vi "引用測試5.vi"() -> ()   [LabVIEW 2015]
uses:
  <vilib>/vision/Measure.llb/Edge Options.ctl
  <vilib>/vision/Measure.llb/Edge Polarity.ctl
  <vilib>/userdefined/High Color/IMAQdx.ctl
  <vilib>/vision/driver/NI_Vision_Acquisition_Software.lvlib
  <vilib>/vision/NI_Vision_Development_Module.lvlib
panel:
  in  "Tab Control":T1(tab)
  in  "邊":T2(ring)
  out "Line Data":cluster{"X":sgl, "Y":sgl, "T":sgl}
  in  "圓":enum16{"Inner to Outer", "Outer to Inner"}(ring)
  out "Ellipse":T3 {"Minor Axis"."Point 2"."Y" format="%.2f"; "Minor Axis"."Point 2"."X" format="%.2f"; "Minor Axis"."Point 1"."Y" format="%.2f"; "Minor Axis"."Point 1"."X" format="%.2f"; "Major Axis"."Point 2"."Y" format="%.2f"; "Major Axis"."Point 2"."X" format="%.2f"; "Major Axis"."Point 1"."Y" format="%.2f"; "Major Axis"."Point 1"."X" format="%.2f"; "Center"."Y" format="%.2f"; "Center"."X" format="%.2f"}
  in  "線":enum16{"Start to End", "End to Start"}(ring)
  out "Location (Pixel)":cluster{"X":sgl, "Y":sgl}
  in  "DieArea":i32=100 min=10
  in  "ShowData":bool
  in  "抓寬度(方向)":T4(ring)=enum."Horizon(Outer to Inner)"
  in  "Settings":T5={"Contrast"=40, "Filter width"=4, "Steepness"=2, "Subsampling Ratio"=5, "Show Search Area"=FALSE, "Show Search Lines"=FALSE, "Show Edges Found"=FALSE, "Show Result"=TRUE}
  out "Distance":sgl
  in  "繪圖":bool
  in  "繪圖ROI資料":T6=enum."Set Data"
  out "Line Profile":T7(graph)
  in  "Session In":T8="cam1"
  in  "Numeric":i32
  in  "重新開圖":bool
  in  "開圖":bool
  in  "動作":enum16{"什麼也不做", "抓邊", "看灰階", "分析光源均勻度", "抓寬度"}(ring)
  out "Mean":sgl format="%#.2f"
  out "Histogram":T9(graph)
  in  "取像":bool
  in  "Edge Options":T10={"Edge Polarity"=0, "Kernel Size"=3, "Width"=3, "Minimum Edge Strength"=10.0, "Interpolation Type"=enum."Bilinear Fixed", "Data Processing Method"=enum."Average"} {"Edge Polarity" items=["All Edges", "Rising Edges", "Falling Edges"]; "Minimum Edge Strength" format="%.2f"; "Width" step=2; "Kernel Size" step=2}
  out "error out":errorcluster
  out "Gradient Information":dbl[][](graph)
  in  "Process":T12(ring)
  in  "Gap":i32=10 min=1 max=300
  in  "stop":bool
  out "Image":T13(plugin-control)
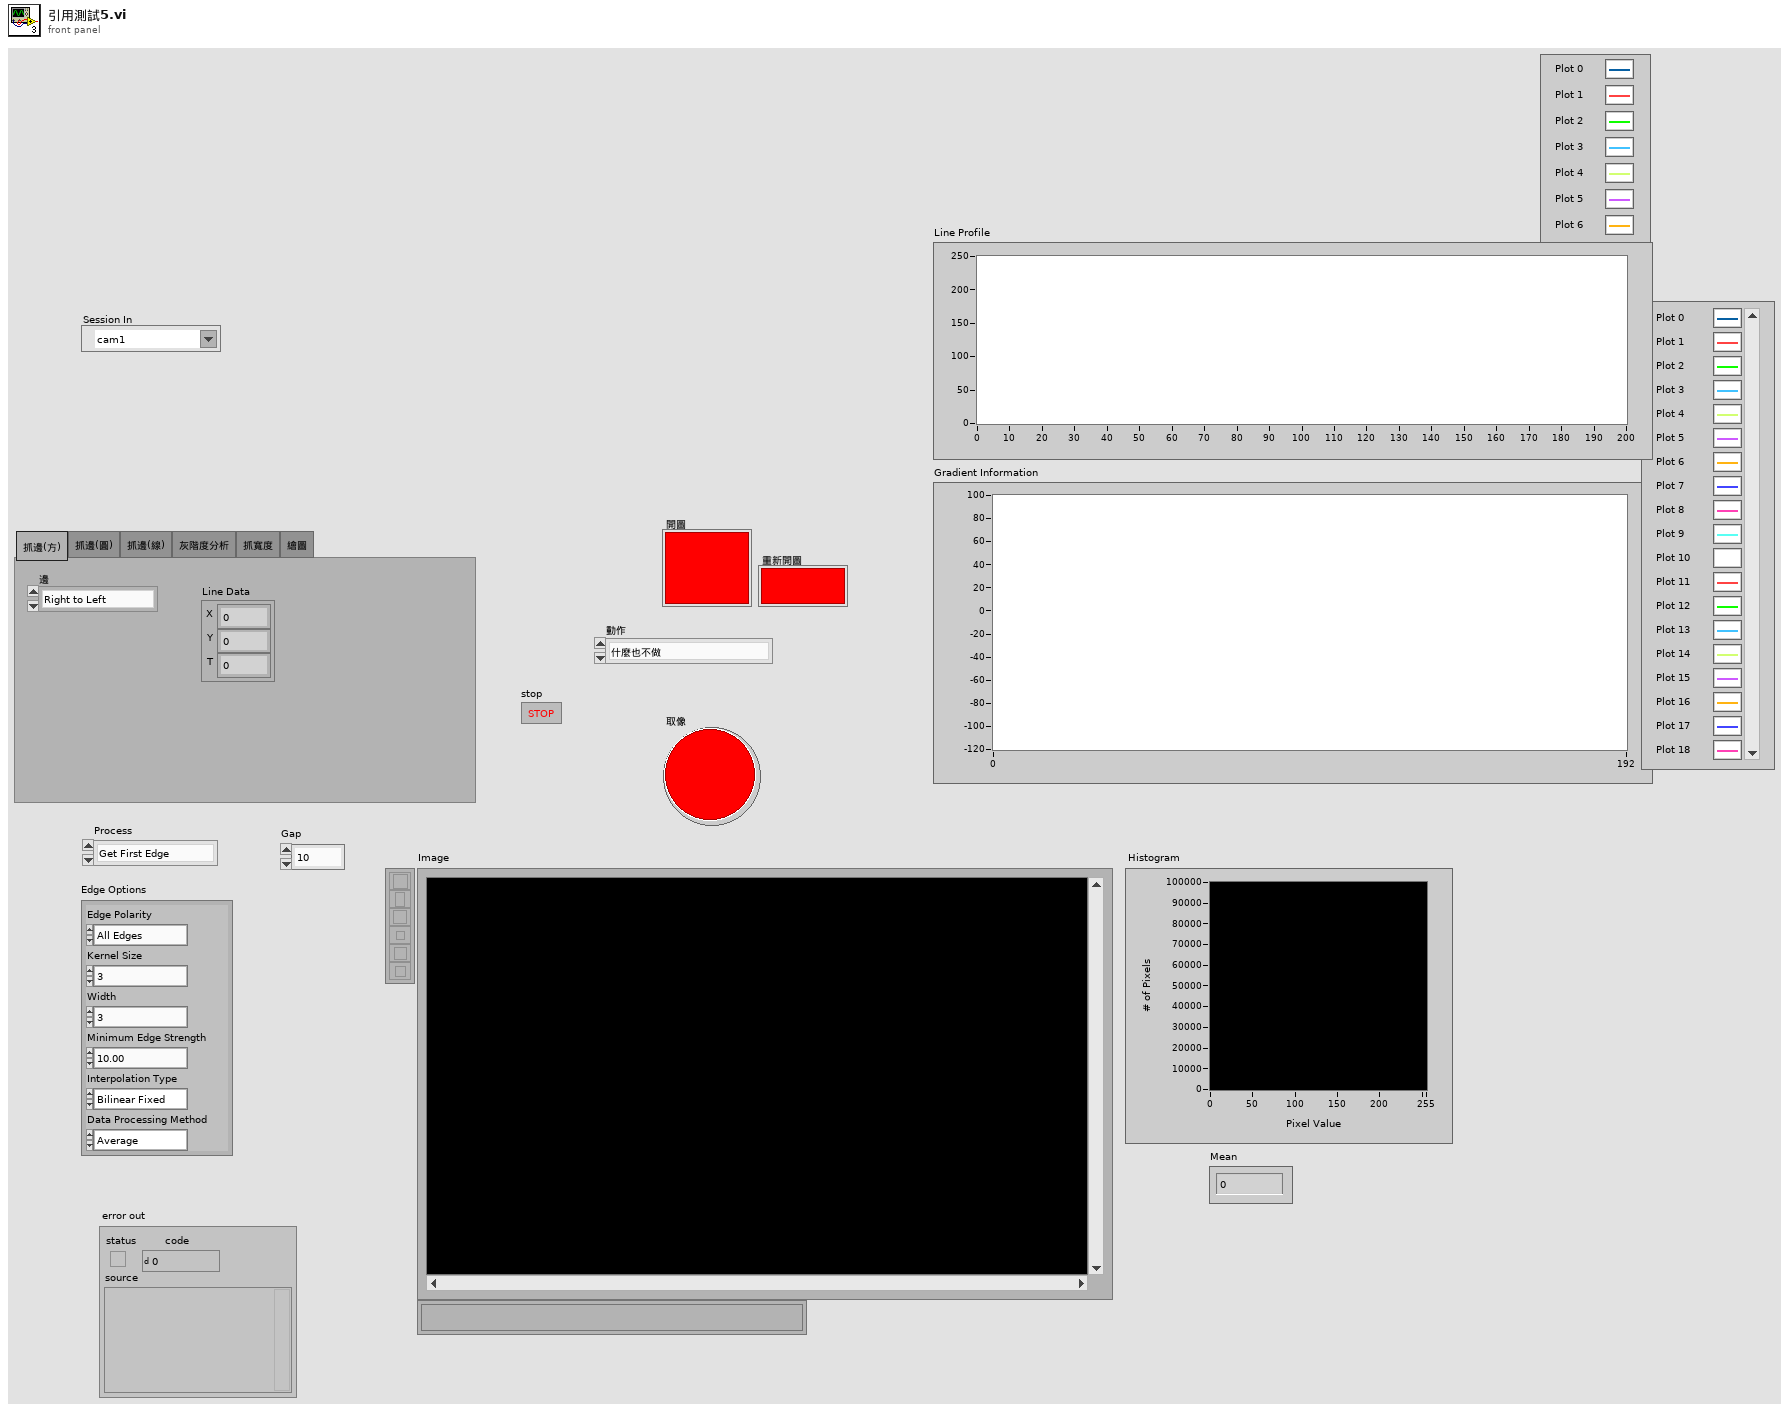
[diagram p1: front panel]
types:
  T1 = enum32{"抓邊(方)", "抓邊(圓)", "抓邊(線)", "灰階度分析", "抓寬度", "繪圖"}
  T2 = enum16{"Right to Left", "Left  to Right", "Up to Down", "Down to Up"}
  T3 = cluster{"Center":cluster{"X":sgl, "Y":sgl}, "Major Axis":cluster{"Point 1":cluster{"X":sgl, "Y":sgl}, "Point 2":cluster{"X":sgl, "Y":sgl}}, "Minor Axis":cluster{"Point 1":cluster{"X":sgl, "Y":sgl}, "Point 2":cluster{"X":sgl, "Y":sgl}}}
  T4 = enum16{"Horizon(Inner to Outer)", "Horizon(Outer to Inner)", "Vertical (Inner to Outer)", "Vertical(Outer to Inner)"}
  T5 = cluster{"Contrast":i32, "Filter width":i32, "Steepness":i32, "Subsampling Ratio":u32, "Show Search Area":bool, "Show Search Lines":bool, "Show Edges Found":bool, "Show Result":bool}
  T6 = typedef "Action_Data.ctl" = enum16{"Initialize", "Get Data", "Set Data", "Delete Data", "Idle"}
  T7 = cluster{"x0":sgl, "dx":sgl, "Pixels Line":sgl[]}[]
  T8 = typedef "IMAQdx.ctl" = refnum<k21>
  T9 = cluster{"Starting Value":sgl, "Incremental Value":sgl, "Histogram":u32[]}
  T10 = typedef "Edge Options.ctl" = cluster{"Edge Polarity":T11, "Kernel Size":u32, "Width":u32, "Minimum Edge Strength":sgl, "Interpolation Type":enum32{"Zero Order", "Bilinear", "Quadratic", "Cubic", "Bilinear Fixed"}, "Data Processing Method":enum32{"Average", "Median"}}
  T11 = typedef "Edge Polarity.ctl" = u32
  T12 = enum16{"Get First Edge", "Get First + Last Edge", "Get All Edges", "Get Best Edge"}
  T13 = typedef "IMAQ Image.ctl" = refnum<image>
  T14 = typedef "IMAQ Rectangle" = cluster{"Left":i32, "Top":i32, "Right":i32, "Bottom":i32, "Rotation":dbl}
  T15 = typedef "ROI Descriptor" = cluster{"Global Rectangle":i32[], "Contours":cluster{"ID":enum32{"External", "Internal"}, "Type":u32, "Coordinates":i32[]}[]}
  T16 = cluster{"Origin":cluster{"X":sgl, "Y":sgl}, "Angle (deg)":sgl, "Axis Reference":u32}
  T17 = typedef "Image Type" = u32
  T18 = cluster{"Global Rectangle":i32[], "Contours":cluster{"Contour Type":u32, "ROI Type":u32, "Points":i32[]}[]}
  T19 = cluster{"Contour Type":u32, "ROI Type":u32, "Points":i32[]}[]
  T20 = cluster{"Contour Type":u32, "ROI Type":u32, "Points":i32[]}
  T21 = enum32{"Zero Order", "Bilinear", "Quadratic", "Cubic", "Bilinear Fixed"}
  T22 = cluster{"邊":enum16{"Right to Left", "Left  to Right", "Up to Down", "Down to Up"}, "動作":enum16{"什麼也不做", "抓邊", "看灰階", "分析光源均勻度", "抓寬度"}, "圓":enum16{"Inner to Outer", "Outer to Inner"}, "Process":enum16{"Get First Edge", "Get First + Last Edge", "Get All Edges", "Get Best Edge"}, "ROI Type":u32, i32, i32, i32, i32, "Gap":i32, i32, i32, i32, i32, "Edge Polarity":T11, "Kernel Size":u32, "Width":u32, "Minimum Edge Strength":sgl, "Interpolation Type":enum32{"Zero Order", "Bilinear", "Quadratic", "Cubic", "Bilinear Fixed"}, "Data Processing Method":enum32{"Average", "Median"}, "DieArea":i32, "ShowData":bool, "線":enum16{"Start to End", "End to Start"}, "抓寬度(方向)":enum16{"Horizon(Inner to Outer)", "Horizon(Outer to Inner)", "Vertical (Inner to Outer)", "Vertical(Outer to Inner)"}, "Contrast":i32, "Filter width":i32, "Steepness":i32, "Subsampling Ratio":u32, "Show Search Area":bool, "Show Search Lines":bool, "Show Edges Found":bool, "Show Result":bool, bool}
  T23 = cluster{"邊":bool, "動作":bool, "圓":bool, "Process":bool, "ROI Type":bool, bool, bool, bool, bool, "Gap":bool, bool, bool, bool, bool, "Edge Polarity":bool, "Kernel Size":bool, "Width":bool, "Minimum Edge Strength":bool, "Interpolation Type":bool, "Data Processing Method":bool, "DieArea":bool, "ShowData":bool, "線":bool, "抓寬度(方向)":bool, "Contrast":bool, "Filter width":bool, "Steepness":bool, "Subsampling Ratio":bool, "Show Search Area":bool, "Show Search Lines":bool, "Show Edges Found":bool, "Show Result":bool, bool}
  T24 = cluster{"Base Reference":cluster{"Origin":cluster{"X":sgl, "Y":sgl}, "Angle (deg)":sgl, "Axis Reference":u32}, "Base Reference":cluster{"Origin":cluster{"X":sgl, "Y":sgl}, "Angle (deg)":sgl, "Axis Reference":u32}}
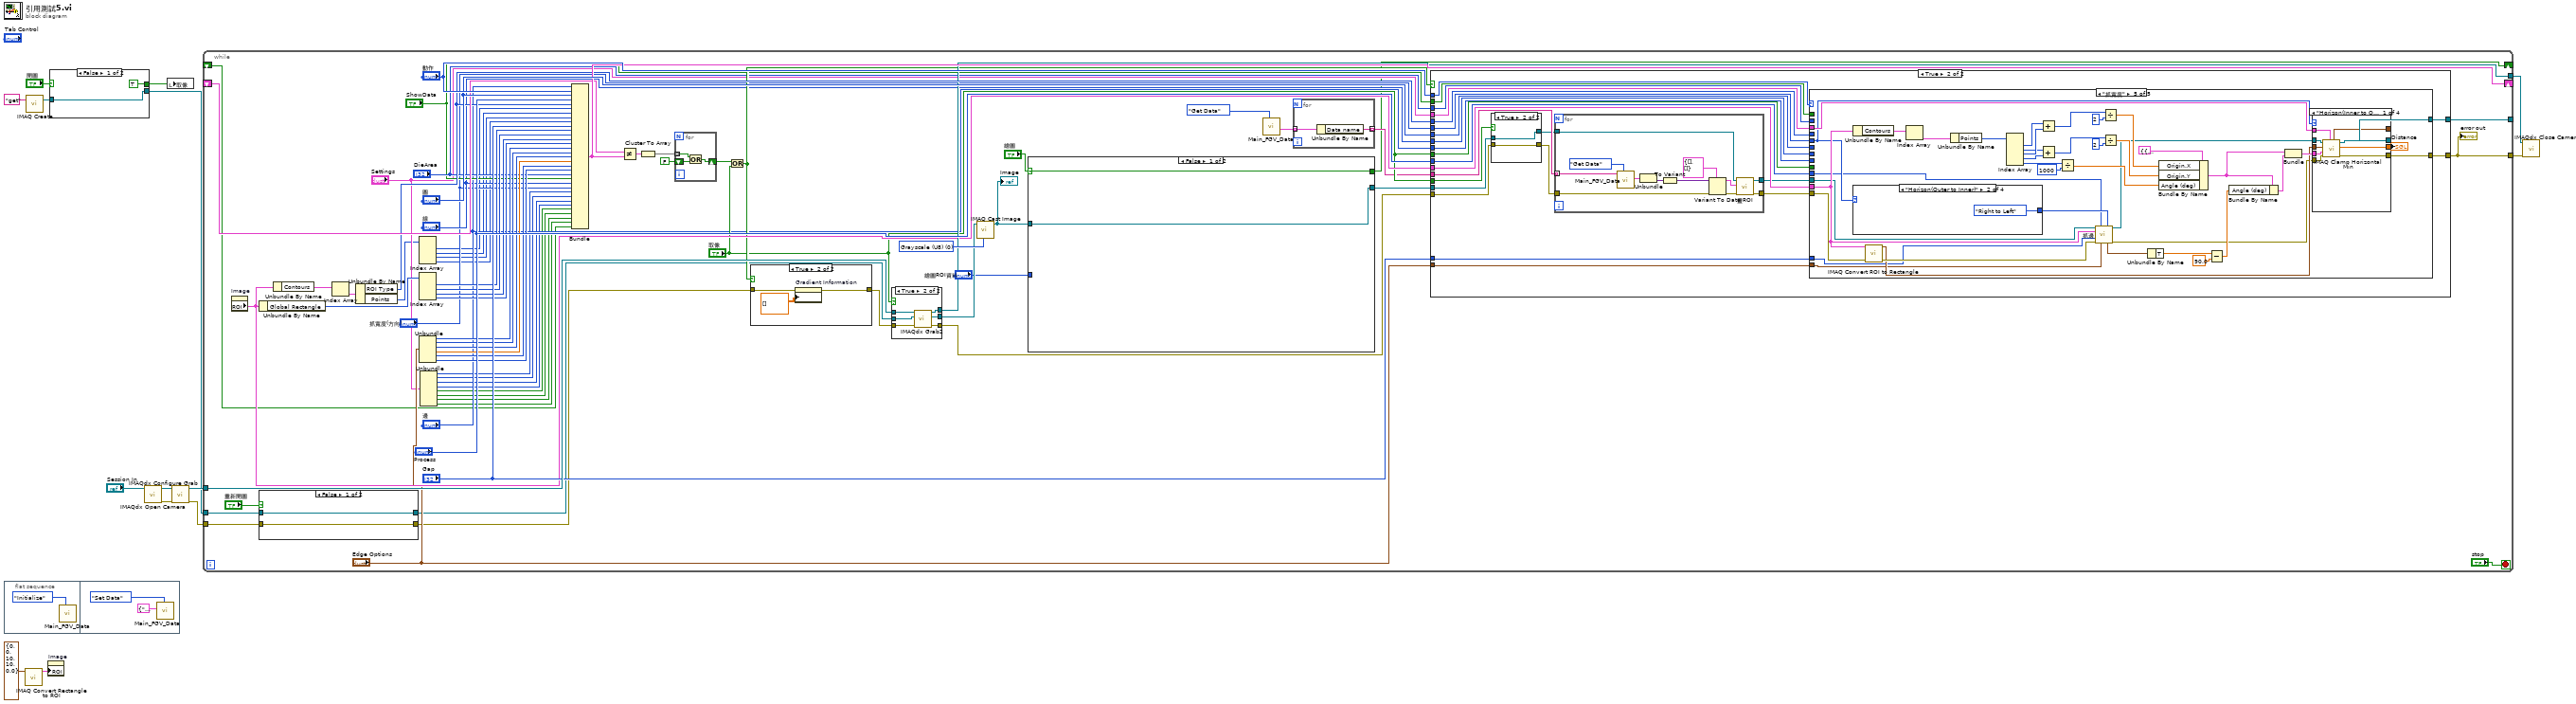
[diagram p0: block diagram]
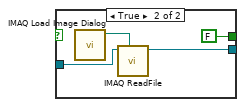
[diagram p2: hidden frame]
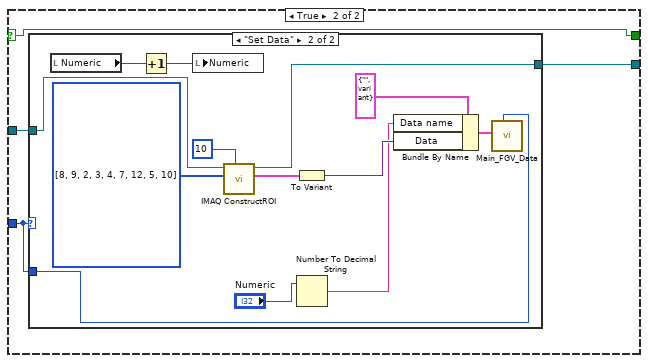
[diagram p3: hidden frame]
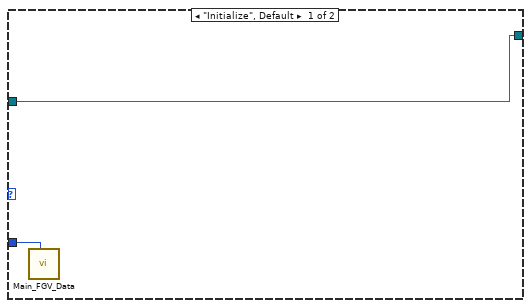
[diagram p4: hidden frame]
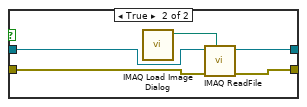
[diagram p5: hidden frame]
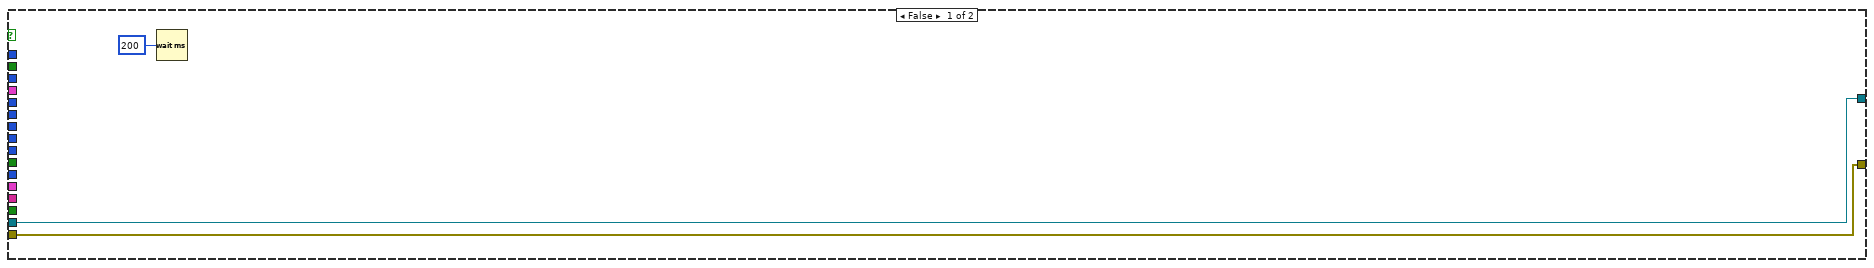
[diagram p7: hidden frame]
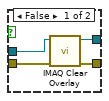
[diagram p8: hidden frame]
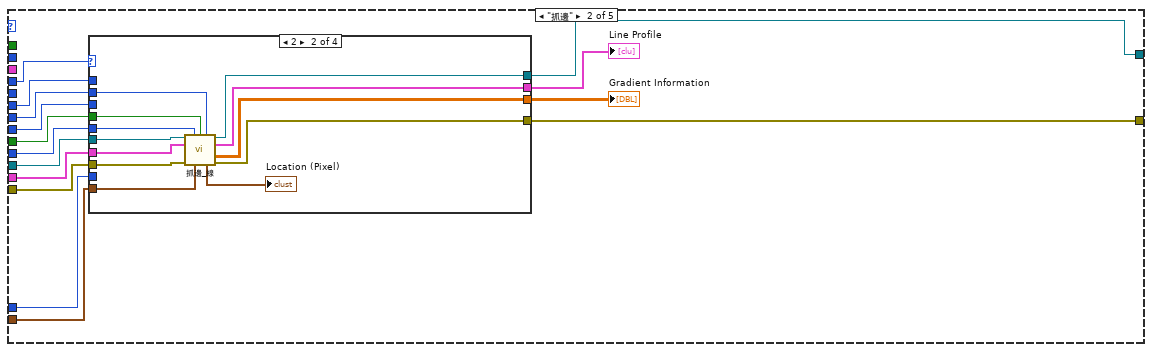
[diagram p10: hidden frame]
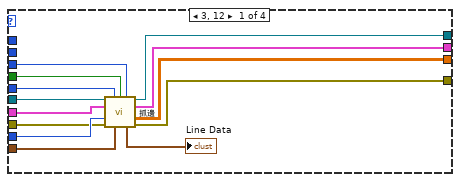
[diagram p11: hidden frame]
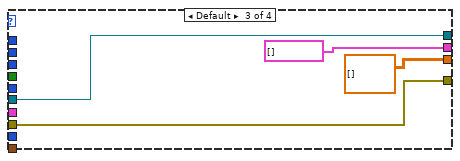
[diagram p12: hidden frame]
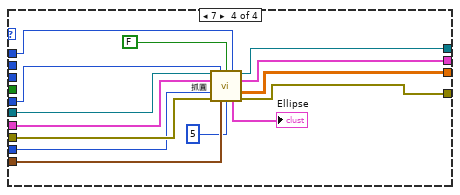
[diagram p13: hidden frame]
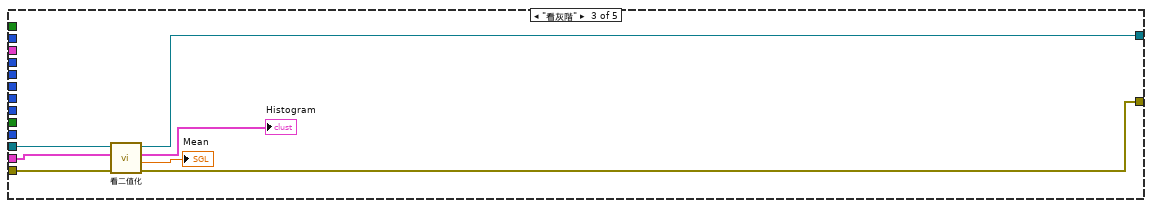
[diagram p14: hidden frame]
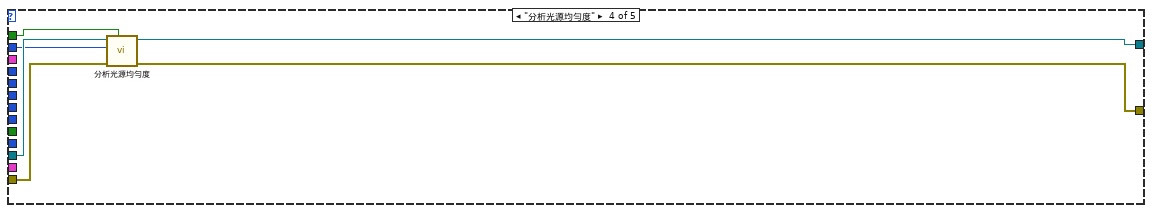
[diagram p15: hidden frame]
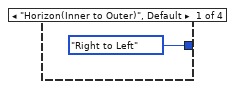
[diagram p16: hidden frame]
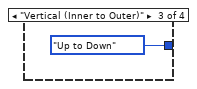
[diagram p17: hidden frame]
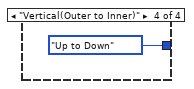
[diagram p18: hidden frame]
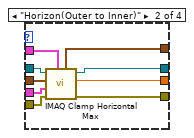
[diagram p19: hidden frame]
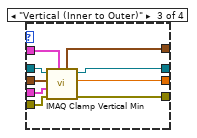
[diagram p20: hidden frame]
diagram:
  n1 = flat-sequence {
    frame #0 {
      n2 = call "Main_FGV_Data.vi"("Action_Data"=Action_Data."Initialize") -> ()  [unwired: 9 in, 2 out]
    }
    frame #1 {
      n3 = call "Main_FGV_Data.vi"("Action_Data"=Action_Data."Set Data", "Data In"=cluster{"Data name":string, "Data":variant} {"Data name"="Oringal", "Data"=variant(cluster{"Global Rectangle":i32[], "Contours":cluster{"ID":enum32{"External", "Internal"}, "Type":u32, "Coordinates":i32[]}[]} {"Global Rectangle"=[0, 959, 2, 960], "Contours"=[{"ID"=enum."External", "Type"=2, "Coordinates"=[0, 959, 1, 959]}]})} ("output cluster 3")) -> ()  [unwired: 8 in, 2 out]
    }
  }
  n4 = call "IMAQ Convert Rectangle to ROI"("Rectangle"=T14 {"Left"=0, "Top"=0, "Right"=10, "Bottom"=10, "Rotation"=0.0}) -> ("ROI Descriptor"=w7:T15)  [unwired: 8 in, 1 out]
  n5 = call "IMAQ Create"("Image Name"="get") -> ("New Image"=w4:T13)  [unwired: 4 in, 1 out]
  n6 = property on="Image" class="ImageControl"("ROI"=w7) -> ()  [unwired: 2 in, 2 out]
  n7 = case shown="False" "開圖" {
    tunnel: [TRUE ("取像") FALSE ("取像")] -> w5
    tunnel: w4 -> [w18 w22]
    tunnel: [w18 w21] -> w3
    frame False {
    }
    frame True {
      n8 = call "IMAQ Load Image Dialog"() -> ("Path"=w20:path)  [unwired: 9 in, 2 out]
      n9 = call "IMAQ ReadFile"("File Path"=w20, "Image"=w22) -> ("Image Out"=w21:T13)  [unwired: 5 in, 4 out]
    }
  }
  n10 = call <vilib>:"IMAQdx Open Camera.vi"("Session In"="Session In") -> ("error out"=w9:errorcluster, "Session Out"=w10:T8)  [unwired: 9 in]
  n11 = local write "取像"(w5) -> ()
  n12 = call <vilib>:"IMAQdx Configure Grab.vi"("error in"=w9, "Session In"=w10) -> ("error out"=w2:errorcluster, "Session Out"=w13:T8)  [unwired: 8 in]
  n13 = while {
    tunnel: w13 -> [w93]
    tunnel: w3 -> [w54]
    tunnel: [w75] -> w12
    tunnel: [w89] -> _
    shift-right: [w84] -> _
    shift-left: _ -> [w83]
    tunnel: w2 -> [w43]
    tunnel: [w31] -> w1
    shift-right: [w30] -> _
    shift-left: _ -> [w29]
    stop <- "stop" stop-if-true
    w91 = T17 0 items=["Grayscale (U8)", "Grayscale (I16)", "Grayscale (SGL)", "Complex (CSG)", "RGB (U32)", "HSL (U32)", "RGB (U64)", "Grayscale (U16)"] ("Image Type")
    n14 = property on="Image" class="ImageControl"() -> ("ROI"=w73:T18)  [unwired: 2 in, 2 out]
    n15 = Unbundle By Name(w73) -> ("Global Rectangle"=w72:i32[])
    n16 = case shown="False" "重新開圖" {
      tunnel: w54 -> [w118 w121]
      tunnel: [w118 w122] -> w53
      tunnel: w43 -> [w117 w120]
      tunnel: [w117 w119] -> w42
      frame False {
      }
      frame True {
        n17 = call "IMAQ Load Image Dialog"() -> ("Path"=w123:path)  [unwired: 9 in, 2 out]
        n18 = call "IMAQ ReadFile"("File Path"=w123, "error in (no error)"=w120, "Image"=w121) -> ("error out"=w119:errorcluster, "Image Out"=w122:T13)  [unwired: 4 in, 3 out]
      }
    }
    n19 = Unbundle By Name(w73) -> ("Contours"=w88:T19)
    n20 = Index Array(array=w88) -> (element=w87:T20)  [unwired: 1 in]
    n21 = Unbundle By Name(w87) -> ("ROI Type"=w77:u32, "Points"=w28:i32[])
    n22 = Index Array(array=w28) -> (element #1=w27:i32, element #2=w26:i32, element #3=w24:i32, element #4=w25:i32)  [unwired: 4 in]
    n23 = Index Array(array=w72) -> (element #1=w71:i32, element #2=w70:i32, element #3=w69:i32, element #4=w68:i32)  [unwired: 4 in]
    n24 = Unbundle("Edge Options") -> ("Edge Polarity"=w65:T11, "Kernel Size"=w64:u32, "Width"=w63:u32, "Minimum Edge Strength"=w62:sgl, "Interpolation Type"=w61:T21, "Data Processing Method"=w60:enum32{"Average", "Median"})
    n25 = Unbundle("Settings") -> ("Contrast"=w40:i32, "Filter width"=w39:i32, "Steepness"=w38:i32, "Subsampling Ratio"=w37:u32, "Show Search Area"=w36:bool, "Show Search Lines"=w35:bool, "Show Edges Found"=w34:bool, "Show Result"=w33:bool)
    n26 = Bundle("邊"="邊", "動作"="動作", "圓"="圓", "Process"="Process", "ROI Type"=w77, w27, w26, w24, w25, "Gap"="Gap", w71, w70, w69, w68, "Edge Polarity"=w65, "Kernel Size"=w64, "Width"=w63, "Minimum Edge Strength"=w62, "Interpolation Type"=w61, "Data Processing Method"=w60, "DieArea"="DieArea", "ShowData"="ShowData", "線"="線", "抓寬度(方向)"="抓寬度(方向)", "Contrast"=w40, "Filter width"=w39, "Steepness"=w38, "Subsampling Ratio"=w37, "Show Search Area"=w36, "Show Search Lines"=w35, "Show Edges Found"=w34, "Show Result"=w33, w29) -> (w84:T22)  [unwired: 1 in]
    n27 = Not Equal?(x=w83, y=w84) -> (x != y?=w76:T23)
    n28 = Cluster To Array(cluster=w76) -> (array=w82:bool[])
    n29 = for {
      tunnel: w82 -> [w130] mode=indexing
      shift-right: [w129] -> w80
      shift-left: FALSE -> [w128]
      n30 = Or(x=w130, y=w128) -> (x .or. y?=w129:bool)
    }
    n31 = Or(x=w80, y="取像") -> (x .or. y?=w67:bool)
    n32 = case shown="True" w67 {
      tunnel: [w124 w126] -> w90
      tunnel: w42 -> [w124 w125]
      frame False {
      }
      frame True {
        n33 = property on="Gradient Information" class="WFChart (strict)"(error in=w125, "History Data"=dbl[][] []) -> (error out=w126:errorcluster)  [unwired: 1 in, 1 out]
      }
    }
    n34 = case shown="True" "取像" {
      tunnel: w93 -> [w331 w337]
      tunnel: w53 -> [w330 w336]
      tunnel: [w331 w335] -> w75
      tunnel: [w330 w334] -> w74
      tunnel: w90 -> [w329 w333]
      tunnel: [w329 w332] -> w47
      frame False {
      }
      frame True {
        n35 = call <vilib>:"IMAQdx Grab2.vi"("error in"=w333, "Image In"=w336, "Session In"=w337) -> ("error out"=w332:errorcluster, "Image Out"=w334:T13, "Session Out"=w335:T8)  [unwired: 5 in, 1 out]
      }
    }
    n36 = call "IMAQ Cast Image"("Image Type"=w91, "Image Src"=w74) -> ("Image Dst Out"=w46:T13)  [unwired: 8 in, 1 out]
    "Image" <- w46
    n37 = case shown="False" "繪圖" {
      selector: "繪圖" -> [w96 w98]
      tunnel: w46 -> [w97 w101]
      tunnel: [w97 w100] -> w45
      tunnel: "繪圖ROI資料" -> [_ w99]
      tunnel: [w96 w98] -> w30
      frame False {
      }
      frame True {
        n38 = case shown="\"Set Data\"" w99 {
          tunnel: w101 -> [w103 w114]
          tunnel: [w103 w112] -> w100
          tunnel: w99 -> [w102 w106]
          frame "Initialize", Default {
            n39 = call "Main_FGV_Data.vi"("Action_Data"=w102) -> ()  [unwired: 9 in, 2 out]
          }
          frame "Set Data" {
            w116 = u32[] [8, 9, 2, 3, 4, 7, 12, 5, 10] items=["No Selection", "Point", "Line", "Rectangle", "Oval", "Polygon", "Freehand Region", "Annulus", "Zoom", "Pan", "Broken Line", "Freehand Line", "Rotated Rectangle"] ("Tools")
            n40 = local read "Numeric"() -> (w108:i32)
            n41 = Increment(x=w108) -> (x+1=w107:i32)
            n42 = local write "Numeric"(w107) -> ()
            n43 = call "IMAQ ConstructROI"("Window Number (-1...15)"=10, "Tools"=w116, "Image"=w114) -> ("ROI Descriptor Out"=w113:T15, "Image Out (duplicate)"=w112:T13)  [unwired: 5 in, 2 out]
            n44 = To Variant(anything=w113) -> (Variant=w111:variant)
            n45 = Number To Decimal String(number="Numeric") -> (decimal integer string=w105:string)  [unwired: 1 in]
            n46 = Bundle By Name(cluster=cluster{"Data name":string, "Data":variant} {"Data name"="", "Data"=variant} ("Data In"), "Data name"=w105, "Data"=w111) -> (w104:cluster{"Data name":string, "Data":variant})
            n47 = call "Main_FGV_Data.vi"("Action_Data"=w106, "Data In"=w104) -> ()  [unwired: 8 in, 2 out]
          }
        }
      }
    }
    n48 = call "Main_FGV_Data.vi"("Action_Data"=Action_Data."Get Data") -> ("Data Array out"=w51:cluster{"Data name":string, "Data":variant}[])  [unwired: 9 in, 1 out]
    n49 = for {
      tunnel: [w95] -> w48 mode=indexing
      tunnel: w51 -> [w94] mode=indexing
      n50 = Unbundle By Name(w94) -> ("Data name"=w95:string)
    }
    n51 = case shown="True" w67 {
      tunnel: "Gap" -> [_ w157]
      tunnel: w47 -> [w133 w142]
      tunnel: "Process" -> [_ w156]
      tunnel: w45 -> [w132 w147]
      tunnel: [w132 w155] -> w89
      tunnel: w73 -> [_ w154]
      tunnel: w77 -> [_ w153]
      tunnel: "Edge Options" -> [_ w152]
      tunnel: [w133 w151] -> w31
      tunnel: "動作" -> [_ w150]
      tunnel: "圓" -> [_ w149]
      tunnel: "取像" -> [_ w148]
      tunnel: "取像" -> [_ w146]
      tunnel: "DieArea" -> [_ w145]
      tunnel: "ShowData" -> [_ w144]
      tunnel: "邊" -> [_ w143]
      tunnel: w48 -> [_ w140]
      tunnel: "線" -> [_ w136]
      tunnel: "抓寬度(方向)" -> [_ w135]
      tunnel: "Settings" -> [_ w134]
      frame False {
        n52 = Wait (ms)(milliseconds to wait=u32 200) -> ()  [unwired: 1 out]
      }
      frame True {
        n53 = case shown="True" w148 {
          tunnel: w147 -> [w172 w175]
          tunnel: [w173 w175] -> w138
          tunnel: w142 -> [w171 w174]
          tunnel: [w170 w174] -> w139
          frame False {
            n54 = call "IMAQ Clear Overlay"("error in (no error)"=w171, "Image"=w172) -> ("error out"=w170:errorcluster, "Image Out"=w173:T13)  [unwired: 8 in]
          }
          frame True {
          }
        }
        n55 = for {
          tunnel: w138 -> [w169]
          tunnel: [w168] -> w137
          tunnel: w139 -> [w159]
          tunnel: [w158] -> w141
          tunnel: w140 -> [w160] mode=indexing
          n56 = call "Main_FGV_Data.vi"("Action_Data"=Action_Data."Get Data", "Data name"=w160) -> ("Data  Out"=w166:cluster{"Data name":string, "Data":variant})  [unwired: 8 in, 1 out]
          n57 = Unbundle(w166) -> ("Data"=w165:variant)  [unwired: 1 out]
          n58 = To Variant(anything=w165) -> (Variant=w164:variant)
          n59 = Variant To Data(error in=w159, type=T15 {"Global Rectangle"=[], "Contours"=[]} ("ROI Descriptor"), Variant=w164) -> (data=w162:T15, error out=w161:errorcluster)
          n60 = call "畫ROI.vi"("error in (no error)"=w161, "ROI In"=w162, "Image In"=w169) -> ("error out"=w158:errorcluster, "Image Out"=w168:T13)  [unwired: 7 in]
        }
        n61 = case shown="\"抓寬度\"" w150 {
          tunnel: w157 -> [_ w192 _ _ w249]
          tunnel: w141 -> [w176 w180 w239 w244 w257]
          tunnel: w149 -> [_ w191 _ _ _]
          tunnel: w156 -> [_ w190 _ _ w251]
          tunnel: w137 -> [w177 w189 w241 w246 w253]
          tunnel: [w177 w188 w242 w247 w288] -> w155
          tunnel: w154 -> [_ w187 w240 _ w258]
          tunnel: w153 -> [_ w186 _ _ _]
          tunnel: w152 -> [_ w185 _ _ w250]
          tunnel: [w176 w183 w236 w248 w286] -> w151
          tunnel: w146 -> [_ w182 _ _ _]
          tunnel: w145 -> [_ _ _ w245 _]
          tunnel: w144 -> [_ _ _ w243 _]
          tunnel: w143 -> [_ w181 _ _ _]
          tunnel: w136 -> [_ w179 _ _ _]
          tunnel: w135 -> [_ _ _ _ w255]
          tunnel: w134 -> [_ _ _ _ w285]
          frame "什麼也不做", Default {
          }
          frame "抓邊" {
            n62 = case shown="2" w186 {
              tunnel: w187 -> [w204 w217 _ w231]
              tunnel: w192 -> [w203 _ _ w232]
              tunnel: w180 -> [w202 w215 w219 w233]
              tunnel: w191 -> [_ _ _ w228]
              tunnel: w190 -> [w197 w212 _ w229]
              tunnel: [w200 w209 dbl[][] [] ("Gradient Information") w235] -> w184
              tunnel: w189 -> [w205 w216 w221 w230]
              tunnel: [w199 w213 w221 w224] -> w188
              tunnel: [w201 w214 w219 w226] -> w183
              tunnel: w185 -> [w198 w208 _ w234]
              tunnel: w182 -> [w196 w211 _ _]
              tunnel: w181 -> [w194 _ _ _]
              tunnel: w179 -> [_ w210 _ _]
              tunnel: [w193 w206 T7 [] ("Line Profile") w222] -> w178
              frame 3, 12 {
                n63 = call "抓邊.vi"("Image In"=w205, "Process"=w197, "Optimized Mode"=w196, "Direction"=w194, "ROI"=w204, "Gap"=w203, "error In"=w202, "Edge Options"=w198) -> ("Image Out"=w199:T13, "Line Profile"=w193:T7, "Gradient Information"=w200:dbl[][], "Line Data"=→"Line Data":cluster{"X":sgl, "Y":sgl, "T":sgl}, "error out"=w201:errorcluster)  [unwired: 3 in]
              }
              frame 2 {
                n64 = call "抓邊_線.vi"("Image In"=w216, "Process"=w212, "Optimized Mode"=w211, "Direction"=w210, "ROI"=w217, "error In"=w215, "Edge Options"=w208) -> ("Image Out"=w213:T13, "Line Profile"=w206:T7, "Gradient Information"=w209:dbl[][], "Location (Pixel)"=→"Location (Pixel)":cluster{"X":sgl, "Y":sgl}, "error out"=w214:errorcluster)  [unwired: 4 in]
              }
              frame Default {
              }
              frame 7 {
                n65 = call "抓圓.vi"("Image In"=w230, "Process"=w229, "Optimized Mode"=FALSE, "Direction"=w228, "ROI"=w231, "Gap"=w232, "error In"=w233, "Edge Options"=w234, "Point Diameter (5)"=u32 5) -> ("Imag e Out"=w224:T13, "Line Profile"=w222:T7, "Gradient Information"=w235:dbl[][], "Ellipse"=→"Ellipse":T3, "error out"=w226:errorcluster)  [unwired: 2 in]
              }
            }
            "Gradient Information" <- w184
            "Line Profile" <- w178
          }
          frame "看灰階" {
            n66 = call "看二值化.vi"("error in (no error)"=w239, "ROI Descriptor"=w240, "Image In"=w241) -> ("error out"=w236:errorcluster, "Mean"=→"Mean":sgl, "Histogram"=→"Histogram":T9, "Image Out"=w242:T13)  [unwired: 4 in, 1 out]
          }
          frame "分析光源均勻度" {
            n67 = call "分析光源均勻度.vi"("ShowData"=w243, "error in (no error)"=w244, "DieArea"=w245, "Image In"=w246) -> ("error out"=w248:errorcluster, "Image"=w247:T13)  [unwired: 6 in]
          }
          frame "抓寬度" {
            n68 = Unbundle By Name(w258) -> ("Contours"=w279:T19)
            n69 = case shown="\"Horizon(Outer to Inner)\"" w255 {
              tunnel: [T2."Right to Left" ("Direction") T2."Right to Left" ("Direction") T2."Up to Down" ("Direction") T2."Up to Down" ("Direction")] -> w254
              frame "Horizon(Inner to Outer)", Default {
              }
              frame "Horizon(Outer to Inner)" {
              }
              frame "Vertical (Inner to Outer)" {
              }
              frame "Vertical(Outer to Inner)" {
              }
            }
            n70 = call "IMAQ Convert ROI to Rectangle"("error in (no error)"=w257, "ROI Descriptor"=w258) -> ("error out"=w263:errorcluster, "Rectangle"=w259:T14)  [unwired: 7 in]
            n71 = Index Array(array=w279) -> (element=w278:T20)  [unwired: 1 in]
            n72 = Unbundle By Name(w278) -> ("Points"=w274:i32[])
            n73 = Index Array(array=w274) -> (element #1=w273:i32, element #2=w271:i32, element #3=w272:i32, element #4=w270:i32, element #5=w261:i32)  [unwired: 5 in]
            n74 = Add(x=w273, y=w272) -> (x+y=w268:i32)
            n75 = Add(x=w271, y=w270) -> (x+y=w269:i32)
            n76 = Divide(x=w261, y=1000) -> (x/y=w276:dbl)
            n77 = call "抓邊.vi"("Image In"=w253, "Process"=w251, "Direction"=w254, "ROI"=w258, "Gap"=w249, "error In"=w263, "Edge Options"=w250) -> ("Image Out"=w252:T13, "Line Data"=w284:cluster{"X":sgl, "Y":sgl, "T":sgl}, "error out"=w256:errorcluster)  [unwired: 4 in, 2 out]
            n78 = Divide(x=w268, y=2) -> (x/y=w265:dbl)
            n79 = Divide(x=w269, y=2) -> (x/y=w264:dbl)
            n80 = Unbundle By Name(w284) -> ("T"=w280:sgl)
            n81 = Bundle By Name(cluster=T16 {"Origin"={"X"=0.0, "Y"=0.0}, "Angle (deg)"=0.0, "Axis Reference"=0} ("Base Reference"), "Origin.X"=w265, "Origin.Y"=w264, "Angle (deg)"=w276) -> (w262:T16)
            n82 = Subtract(x=w280, y=sgl 90.0) -> (x-y=w275:sgl)
            n83 = Bundle By Name(cluster=w262, "Angle (deg)"=w275) -> (w282:T16)
            n84 = Bundle("Base Reference"=w262, "Base Reference"=w282) -> (w260:T24)  [unwired: 1 in]
            n85 = case shown="\"Horizon(Inner to Outer)\", Default" w255 {
              tunnel: w252 -> [w301 w310 w318 w326]
              tunnel: [w300 w307 w316 w325] -> w288
              tunnel: w259 -> [w299 w308 w319 w327]
              tunnel: w256 -> [w298 w309 w317 w328]
              tunnel: [w297 w306 w315 w324] -> w287
              tunnel: [w296 w305 w314 w323] -> w286
              tunnel: w285 -> [w294 w304 w313 w322]
              tunnel: [w295 w303 w312 w321] -> _
              tunnel: w260 -> [w293 w302 w311 w320]
              frame "Horizon(Inner to Outer)", Default {
                n86 = call "IMAQ Clamp Horizontal Min"("Settings"=w294, "error in (no error)"=w298, "Coordinate System"=w293, "Rectangle"=w299, "Image"=w301) -> ("error out"=w296:errorcluster, "Distance"=w297:sgl, "Image Out"=w300:T13, "Edge Coordinates"=w295:cluster{"X":sgl, "Y":sgl}[])  [unwired: 2 in, 1 out]
              }
              frame "Horizon(Outer to Inner)" {
                n87 = call "IMAQ Clamp Horizontal Max"("Settings"=w304, "error in (no error)"=w309, "Coordinate System"=w302, "Rectangle"=w308, "Image"=w310) -> ("error out"=w305:errorcluster, "Distance"=w306:sgl, "Image Out"=w307:T13, "Edge Coordinates"=w303:cluster{"X":sgl, "Y":sgl}[])  [unwired: 2 in, 1 out]
              }
              frame "Vertical (Inner to Outer)" {
                n88 = call "IMAQ Clamp Vertical Min"("Settings"=w313, "error in (no error)"=w317, "Coordinate System"=w311, "Rectangle"=w319, "Image"=w318) -> ("error out"=w314:errorcluster, "Distance"=w315:sgl, "Image Out"=w316:T13, "Edge Coordinates"=w312:cluster{"X":sgl, "Y":sgl}[])  [unwired: 2 in, 1 out]
              }
              frame "Vertical(Outer to Inner)" {
                n89 = call "IMAQ Clamp Vertical Max"("Settings"=w322, "error in (no error)"=w328, "Coordinate System"=w320, "Rectangle"=w327, "Image"=w326) -> ("error out"=w323:errorcluster, "Distance"=w324:sgl, "Image Out"=w325:T13, "Edge Coordinates"=w321:cluster{"X":sgl, "Y":sgl}[])  [unwired: 2 in, 1 out]
              }
            }
            "Distance" <- w287
          }
        }
      }
    }
    "error out" <- w31
  }
  n90 = call <vilib>:"IMAQdx Close Camera.vi"("error in"=w1, "Session In"=w12) -> ()  [unwired: 9 in, 1 out]
